vi "AI data calculation.vi"(0 "Sensor raw":dbl=0.00395, 1 "NTC raw":dbl=0.00395, 2 "U15 raw":dbl=0.00395, 3 "U48 raw":dbl=0.00395, 4 "Isol raw":dbl=0.00395, 5 "Temp raw":dbl=0.00395) -> (11 "NTC ellenállás elvárt":dbl, 13 "Hõmérséklet":dbl, 14 "Sensor ellenállás":dbl, 15 "NTC ellenállás":dbl, 16 "NTC Hõmérséklet számolt":dbl, 17 "15V":dbl, 18 "48V":dbl, 19 "Szigetelési ellenállás":dbl)   [LabVIEW 2014]
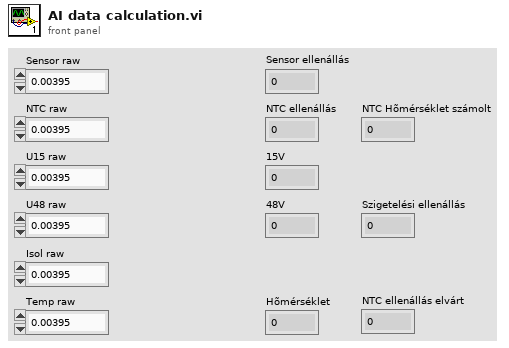
[diagram p1: front panel]
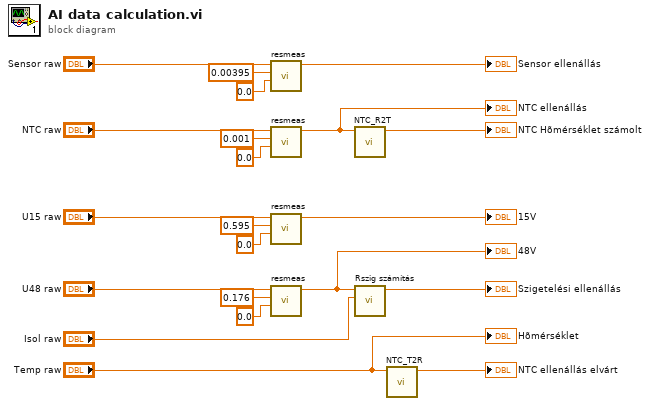
[diagram p0: block diagram]
diagram:
  n1 = call "resmeas.vi"("Rc"=0.0, "Im"=0.00395, "Um"="Sensor raw") -> ("Rm"=→"Sensor ellenállás":dbl)  [unwired: 8 in]
  n2 = call "resmeas.vi"("Rc"=0.0, "Im"=0.001, "Um"="NTC raw") -> ("Rm"=w9:dbl)  [unwired: 8 in]
  "NTC ellenállás" <- w9
  n3 = call "resmeas.vi"("Rc"=0.0, "Im"=0.595, "Um"="U15 raw") -> ("Rm"=→"15V":dbl)  [unwired: 8 in]
  n4 = call "resmeas.vi"("Rc"=0.0, "Im"=0.176, "Um"="U48 raw") -> ("Rm"=w4:dbl)  [unwired: 8 in]
  "48V" <- w4
  n5 = call "NTC_R2T.vi"("Resistance"=w9) -> ("Temperature"=→"NTC Hõmérséklet számolt":dbl)  [unwired: 10 in]
  n6 = call "Rszig számítás.vi"("UIsol"="Isol raw", "U48"=w4) -> ("Rszig"=→"Szigetelési ellenállás":dbl)  [unwired: 9 in]
  n7 = call "NTC_T2R.vi"("Temperature"="Temp raw") -> ("Resistance"=→"NTC ellenállás elvárt":dbl)  [unwired: 10 in]
  "Hõmérséklet" <- "Temp raw"
